vi "Align and Distribute.vi"(6 "Variant in":variant, 7 "Shift Pressed?":bool, 8 "error in (no error)":errorcluster, 10 "QD Combo Box Ref":refnum<vi>, 11 "QD Launch VI Ref":refnum<vi>) -> (0 "error out":errorcluster, 4 "Variant out":variant)   [LabVIEW 2012, in "Align and Distribute.lvlib"]
doc: "PLUGIN_DESCRIPTION: Aligns selected items to the right, left, top or bottom or by horizontal or vertical centers by pressing r, l, t, b, h or v.\n\nPLUGIN_DEFAULT_SHORTCUT: A"
uses:
  Align and Distribute.lvlib
panel:
  # "Do not change the connector pane of this VI."
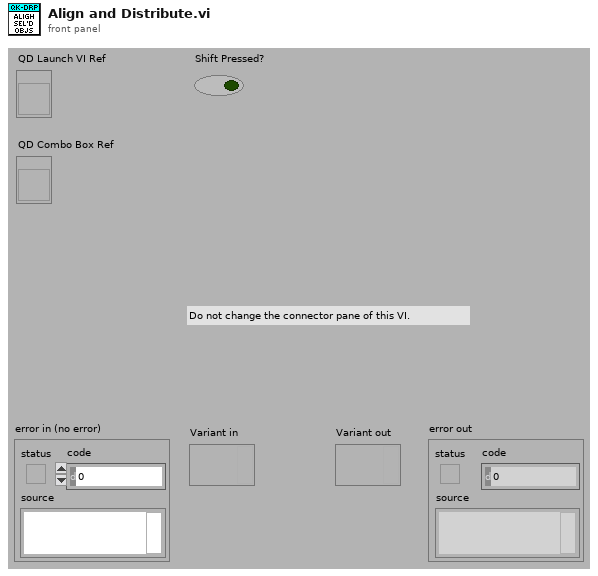
[diagram p1: front panel]
types:
  T1 = enum32{"Top Edges", "Vertical Centers", "Bottom Edges", "Vertical Gap", "Vertical Compress", "Left Edges", "Horizontal Centers", "Right Edges", "Horizontal Gap", "Horizontal Compress"}
  T2 = enum32{"Top Edges", "Vertical Centers", "Bottom Edges", "Left Edges", "Horizontal Centers", "Right Edges"}
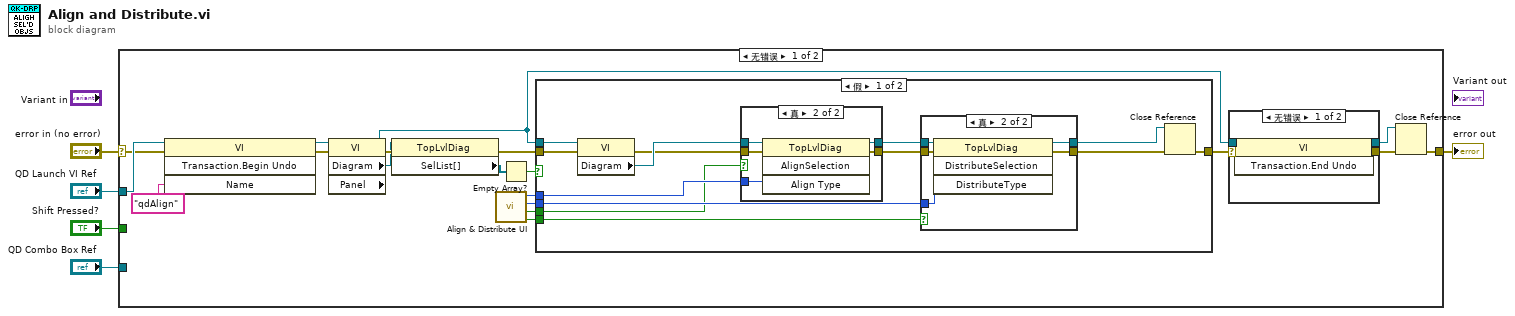
[diagram p0: block diagram]
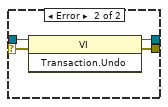
[diagram p2: hidden frame]
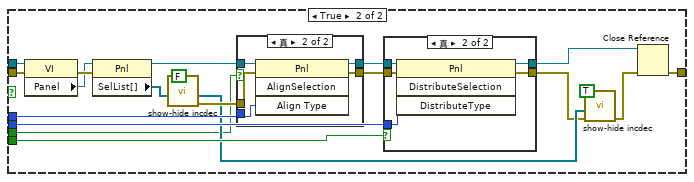
[diagram p5: hidden frame]
diagram:
  n1 = case shown="无错误" "error in (no error)" {
    selector: "error in (no error)" -> [w17 w94]
    tunnel: [w20 w94] -> w4
    tunnel: "QD Launch VI Ref" -> [w19 _]
    tunnel: "Shift Pressed?" -> [_ _]
    tunnel: "QD Combo Box Ref" -> [_ _]
    frame No Error {
      n2 = invoke class="VI" method="Transaction.Begin Undo"(reference=w19, error in=w17, "Name"="qdAlign") -> (reference out=w18:refnum<vi>, error out=w16:errorcluster)  [unwired: 1 in, 2 out]
      n3 = property class="VI" props=["Diagram", "Panel"](reference=w18, error in=w16) -> (reference out=w13:refnum<vi>, error out=w24:errorcluster, "Diagram"=w23:refnum<vi>)  [unwired: 1 out]
      n4 = property class="TopLvlDiag"(reference=w23, error in=w24) -> (error out=w21:errorcluster, "SelList[]"=w8:refnum<vi>[])  [unwired: 1 out]
      n5 = call "Align & Distribute UI.vi"() -> ("Distribute Type valid?"=w7:bool, "Align Type valid?"=w6:bool, "Distribute Type"=w10:T1, "Align Type"=w11:T2)  [unwired: 8 in]
      n6 = Empty Array?(array=w8) -> (empty?=w22:bool)
      n7 = case shown="假" w22 {
        tunnel: w21 -> [w44 w79]
        tunnel: w13 -> [w43 w78]
        tunnel: [w45 w77] -> w9
        tunnel: w11 -> [w40 w76]
        tunnel: w7 -> [w35 w72]
        tunnel: w10 -> [w34 w71]
        tunnel: w6 -> [w33 w60]
        frame False {
          n8 = property class="VI"(reference=w43, error in=w44) -> (error out=w41:errorcluster, "Diagram"=w42:refnum<vi>)  [unwired: 1 out]
          n9 = case shown="真" w33 {
            tunnel: w42 -> [w47 w52]
            tunnel: w41 -> [w46 w51]
            tunnel: w40 -> [_ w50]
            tunnel: [w46 w49] -> w39
            tunnel: [w47 w48] -> w38
            frame False {
            }
            frame True {
              n10 = invoke class="TopLvlDiag" method="AlignSelection"(reference=w52, error in=w51, "Align Type"=w50) -> (reference out=w48:refnum<vi>, error out=w49:errorcluster)  [unwired: 1 in, 2 out]
            }
          }
          n11 = case shown="真" w35 {
            tunnel: w39 -> [w54 w59]
            tunnel: w38 -> [w53 w58]
            tunnel: [w53 w57] -> w37
            tunnel: [w54 w56] -> w36
            tunnel: w34 -> [_ w55]
            frame False {
            }
            frame True {
              n12 = invoke class="TopLvlDiag" method="DistributeSelection"(reference=w58, error in=w59, "DistributeType"=w55) -> (reference out=w57:refnum<vi>, error out=w56:errorcluster)  [unwired: 1 in, 2 out]
            }
          }
          n13 = Close Reference(reference=w37, error in (no error)=w36) -> (error out=w45:errorcluster)
        }
        frame True {
          n14 = property class="VI"(reference=w78, error in=w79) -> (error out=w68:errorcluster, "Panel"=w67:refnum<vi>)  [unwired: 1 out]
          n15 = property class="Pnl"(reference=w67, error in=w68) -> (reference out=w66:refnum<vi>, "SelList[]"=w69:refnum<vi>[])  [unwired: 1 out]
          n16 = call "show-hide incdec.vi"("Show?"=FALSE, "SelList[]"=w69) -> ("error out"=w65:errorcluster, "SelList[] out"=w63:refnum<vi>[])  [unwired: 8 in]
          n17 = case shown="真" w60 {
            tunnel: w76 -> [_ w86]
            tunnel: [w80 w85] -> w75
            tunnel: [w81 w84] -> w74
            tunnel: w66 -> [w81 w83]
            tunnel: w65 -> [w80 w82]
            frame False {
            }
            frame True {
              n18 = invoke class="Pnl" method="AlignSelection"(reference=w83, error in=w82, "Align Type"=w86) -> (reference out=w84:refnum<vi>, error out=w85:errorcluster)  [unwired: 1 in, 2 out]
            }
          }
          n19 = case shown="真" w72 {
            tunnel: w75 -> [w88 w93]
            tunnel: w74 -> [w87 w92]
            tunnel: [w87 w91] -> w73
            tunnel: [w88 w90] -> w62
            tunnel: w71 -> [_ w89]
            frame False {
            }
            frame True {
              n20 = invoke class="Pnl" method="DistributeSelection"(reference=w92, error in=w93, "DistributeType"=w89) -> (reference out=w91:refnum<vi>, error out=w90:errorcluster)  [unwired: 1 in, 2 out]
            }
          }
          n21 = call "show-hide incdec.vi"("Show?"=TRUE, "error in"=w62, "SelList[]"=w63) -> ("error out"=w61:errorcluster)  [unwired: 7 in, 1 out]
          n22 = Close Reference(reference=w73, error in (no error)=w61) -> (error out=w77:errorcluster)
        }
      }
      n23 = case shown="无错误" w9 {
        selector: w9 -> [w25 w32]
        tunnel: [w28 w31] -> w14
        tunnel: w13 -> [w27 w30]
        tunnel: [w26 w29] -> w12
        frame No Error {
          n24 = invoke class="VI" method="Transaction.End Undo"(reference=w27, error in=w25) -> (reference out=w26:refnum<vi>, error out=w28:errorcluster)  [unwired: 1 in, 1 out]
        }
        frame Error {
          n25 = invoke class="VI" method="Transaction.Undo"(reference=w30, error in=w32) -> (reference out=w29:refnum<vi>, error out=w31:errorcluster)  [unwired: 1 in, 1 out]
        }
      }
      n26 = Close Reference(reference=w12, error in (no error)=w14) -> (error out=w20:errorcluster)
    }
    frame Error {
    }
  }
  "error out" <- w4
